vi "Get TDMS channel with scaling.vi"(6 "Samples per read":i64=1000000, 7 "Clip/desimate":T1={"Clip time"=FALSE, "Tiime 0"=0.0, "Time 1"=0.0, "Maximum data points"=1, "Decimation method"=enum."Min-Max"}, 8 "error in":errorcluster, 9 "Channel name":string, 10 "group name":string, 11 "tdms file":refnum<k34>) -> (0 "error out":errorcluster, 1 "output waveform":waveform(sgl), 3 "tdms file out":refnum<k34>)   [LabVIEW 2015]
uses:
  Controls/Data reduction.ctl
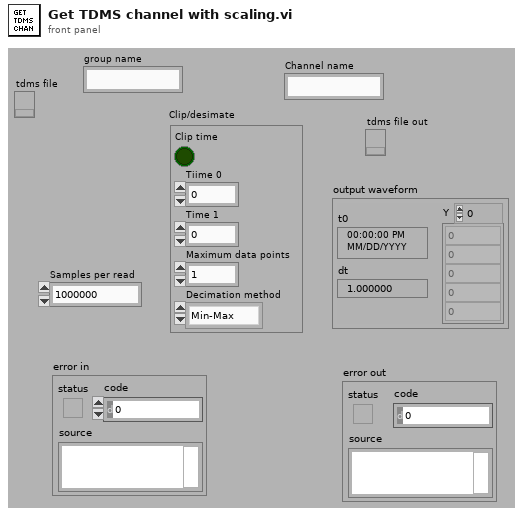
[diagram p1: front panel]
types:
  T1 = typedef "Data reduction.ctl" = cluster{"Clip time":bool, "Tiime 0":dbl, "Time 1":dbl, "Maximum data points":i32, "Decimation method":enum16{"coerce", "linear", "spline", "Min-Max", "Average"}}
  T2 = enum16{"coerce", "linear", "spline", "Min-Max", "Average"}
  T3 = typedef "TDMS channel info.ctl" = cluster{"t0":timestamp, "dt":dbl, "Channel length":i64}
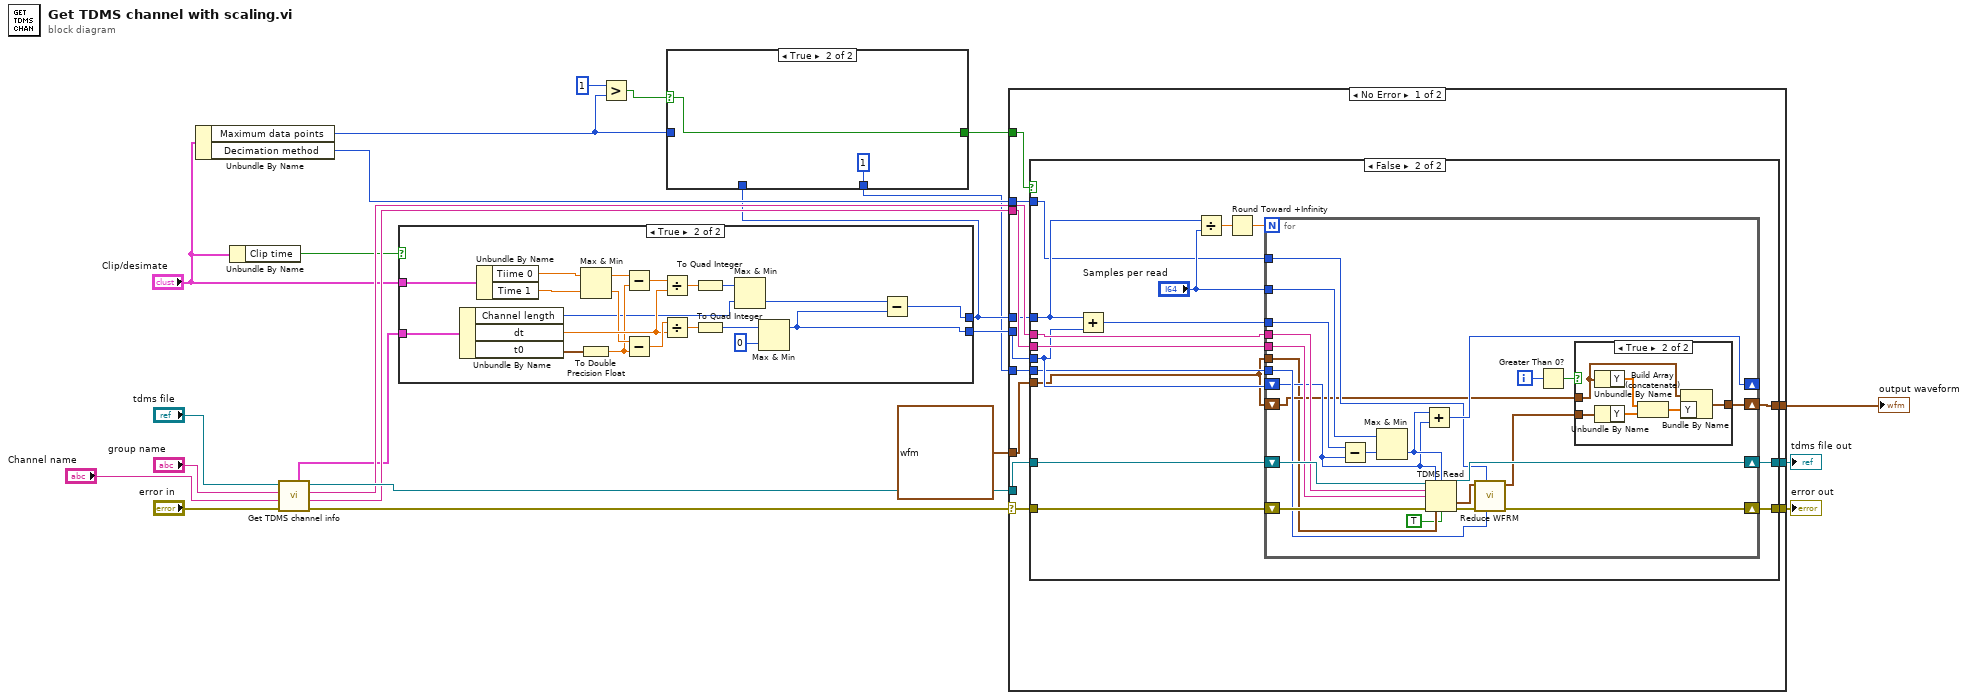
[diagram p0: block diagram]
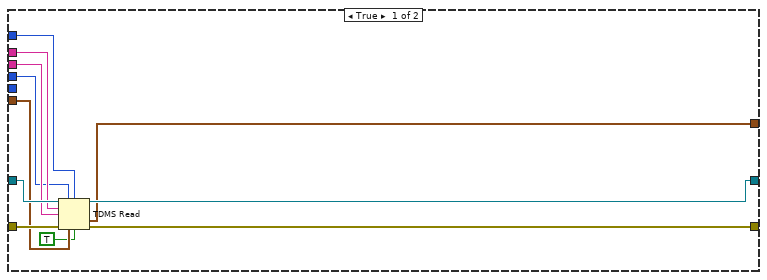
[diagram p2: hidden frame]
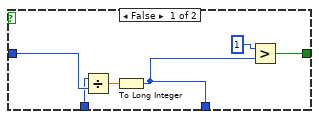
[diagram p5: hidden frame]
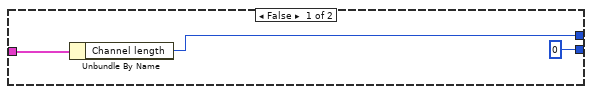
[diagram p6: hidden frame]
diagram:
  n1 = Unbundle By Name("Clip/desimate") -> ("Maximum data points"=w3:i32, "Decimation method"=w11:T2)
  n2 = Unbundle By Name("Clip/desimate") -> ("Clip time"=w8:bool)
  n3 = call "Get TDMS channel info.vi"("error in"="error in", "Channel name"="Channel name", "group name"="group name", "tdms file"="tdms file") -> ("error out"=w1:errorcluster, "channel name out"=w17:string, "group name out"=w18:string, "tdms file out"=w19:refnum<k34>, "TDMS channel info"=w7:T3)  [unwired: 3 in]
  n4 = case shown="True" w8 {
    tunnel: w7 -> [w25 w46]
    tunnel: [i64 0 ("offset (0)") w29] -> w14
    tunnel: [w24 w28] -> w5
    tunnel: "Clip/desimate" -> [_ w37]
    frame False {
      n5 = Unbundle By Name(w25) -> ("Channel length"=w24:i64)
    }
    frame True {
      n6 = Unbundle By Name(w46) -> ("Channel length"=w27:i64, "dt"=w38:dbl, "t0"=w33:timestamp)
      n7 = Unbundle By Name(w37) -> ("Tiime 0"=w36:dbl, "Time 1"=w35:dbl)
      n8 = Max & Min(x=w36, y=w35) -> (max(x,y)=w34:dbl, min(x,y)=w32:dbl)
      n9 = To Double Precision Float(number=w33) -> (double precision float=w31:dbl)
      n10 = Subtract(x=w34, y=w31) -> (x-y=w45:dbl)
      n11 = Subtract(x=w32, y=w31) -> (x-y=w44:dbl)
      n12 = Divide(x=w45, y=w38) -> (x/y=w43:dbl)
      n13 = Divide(x=w44, y=w38) -> (x/y=w40:dbl)
      n14 = To Quad Integer(1:w43) -> (0:w42:i64)
      n15 = To Quad Integer(1:w40) -> (0:w41:i64)
      n16 = Max & Min(x=w42, y=w27) -> (min(x,y)=w30:i64)  [unwired: 1 out]
      n17 = Max & Min(x=w41, y=i64 0) -> (max(x,y)=w29:i64)  [unwired: 1 out]
      n18 = Subtract(x=w30, y=w29) -> (x-y=w28:i64)
    }
  }
  n19 = Greater?(x=1 ("y"), y=w3) -> (0:w6:bool)
  n20 = case shown="True" w6 {
    selector: w6 -> [_ w54]
    tunnel: [w52 w54] -> w13
    tunnel: w3 -> [w49 _]
    tunnel: w5 -> [w48 _]
    tunnel: [w47 1] -> w2
    frame False {
      n21 = Divide(x=w48, y=w49) -> (x/y=w50:dbl)
      n22 = To Long Integer(number=w50) -> (32bit integer=w47:i32)
      n23 = Greater?(x=1 ("y"), y=w47) -> (0:w52:bool)
    }
    frame True {
    }
  }
  n24 = case shown="No Error" w1 {
    selector: w1 -> [w55 w127]
    tunnel: w19 -> [w67 w126]
    tunnel: w18 -> [w66 _]
    tunnel: w17 -> [w65 _]
    tunnel: [w64 w126] -> w16
    tunnel: [w63 w127] -> w15
    tunnel: w14 -> [w62 _]
    tunnel: w13 -> [w61 _]
    tunnel: [w60 w125] -> w12
    tunnel: w11 -> [w59 _]
    tunnel: waveform(sgl) {"t0"=timestamp(0 s since 1904-01-01), "dt"=1.0, "Y"=[]} ("Waveform out") -> [w58 w125]
    tunnel: w5 -> [w57 _]
    tunnel: w2 -> [w56 _]
    frame No Error {
      n25 = case shown="False" w61 {
        tunnel: w55 -> [w78 w94]
        tunnel: w67 -> [w77 w93]
        tunnel: w66 -> [w76 w92]
        tunnel: w65 -> [w75 w91]
        tunnel: [w74 w90] -> w64
        tunnel: [w73 w89] -> w63
        tunnel: w62 -> [w72 w85]
        tunnel: w57 -> [w71 w84]
        tunnel: [w70 w88] -> w60
        tunnel: w56 -> [_ w82]
        tunnel: w59 -> [_ w80]
        tunnel: w58 -> [w69 w79]
        frame True {
          n26 = TDMS Read(0:w77, 1:w72, 2:w71, 5:w76, 7:w75, 11:w78, 12:w69, 13:TRUE ("return channels in file order? (F)")) -> (4:w74:refnum<k34>, 10:w70:waveform(sgl), 15:w73:errorcluster)  [unwired: 3 out]
        }
        frame False {
          n27 = Add(x=w84, y=w85) -> (x+y=w83:i64)
          n28 = Divide(x=w84, y="Samples per read") -> (x/y=w87:dbl)
          n29 = Round Toward +Infinity(x=w87) -> (ceil(x): smallest int >= x=w81:dbl)
          n30 = for {
            N: w81 -> [_]
            tunnel: w92 -> [w115]
            tunnel: w91 -> [w114]
            shift-right: [w113] -> w90
            shift-left: w93 -> [w116]
            shift-right: [w102] -> w89
            shift-left: w94 -> [w117]
            shift-right: [w104] -> _
            shift-left: w85 -> [w105]
            tunnel: "Samples per read" -> [w112]
            tunnel: w83 -> [w111]
            tunnel: w82 -> [w107]
            shift-right: [w101] -> w88
            shift-left: w79 -> [w97]
            tunnel: w80 -> [w100]
            tunnel: w79 -> [w96]
            i -> [w99]
            n31 = Subtract(x=w111, y=w105) -> (x-y=w110:i64)
            n32 = Max & Min(x=w112, y=w110) -> (min(x,y)=w106:i64)  [unwired: 1 out]
            n33 = Add(x=w106, y=w105) -> (x+y=w104:i64)
            n34 = TDMS Read(0:w116, 1:w105, 2:w106, 5:w115, 7:w114, 11:w117, 12:w96, 13:TRUE ("return channels in file order? (F)")) -> (4:w113:refnum<k34>, 10:w108:waveform(sgl), 15:w109:errorcluster)  [unwired: 3 out]
            n35 = call "Reduce WFRM.vi"("decimation factor"=w107, "Decimation method"=w100, "error in (no error)"=w109, "Waveform"=w108) -> ("error out"=w102:errorcluster, "Waveform out"=w103:waveform(sgl))  [unwired: 6 in]
            n36 = Greater Than 0?(x=w99) -> (x > 0?=w98:bool)
            n37 = case shown="True" w98 {
              tunnel: w103 -> [w118 w120]
              tunnel: [w118 w121] -> w101
              tunnel: w97 -> [_ w119]
              frame False {
              }
              frame True {
                n38 = Unbundle By Name(w119) -> ("Y"=w123:sgl[])
                n39 = Unbundle By Name(w120) -> ("Y"=w124:sgl[])
                n40 = Build Array (concatenate)(w123, w124) -> (w122:sgl[])
                n41 = Bundle By Name(cluster=w119, "Y"=w122) -> (w121:waveform(sgl))
              }
            }
          }
        }
      }
    }
    frame Error {
    }
  }
  "tdms file out" <- w16
  "error out" <- w15
  "output waveform" <- w12
